vi "nanocal -- nuclear schottky fit V5.vi"() -> ()   [LabVIEW 2020] (continued)
__sam_\" ->   <|    \"ζ\" -> 0.023098882919   ,  \"τ1\" -> 0.017709986922   ,  \"τS\" -> 0.038881575014   ,  \"τN\" -> 0.000747654909   ,  \"τC\" -> 0.003803962289   ,  \"κ0\" -> 0.000000003538   ,  \"mm1\" -> 0.000078528513   ,  \"mm2\" -> 0.017209583260   ,  \"mm3\" -> 0.044770458303   ,  \"T\" -> 0.530000000000   ,  \"B\" -> 5.000000000000   ,  \"θ\" -> 90.000000000000   ,  \"Reoff\" -> -1599397.590361446140   ,  \"Imoff\" -> 0.000000000000    |>   , \r\"IDS0344_210904_RAW_cal__ref_\" ->   <|    \"ζ\" -> 0.030262302634   ,  \"τ1\" -> 0.017398280529   ,  \"τS\" -> 0.027078056707   ,  \"τN\" -> 0.000382363637   ,  \"τC\" -> 0.002680781698   ,  \"κ0\" -> 0.000000003878   ,  \"mm1\" -> 0.000072009464   ,  \"mm2\" -> 0.016908620237   ,  \"mm3\" -> 0.031389868421   ,  \"T\" -> 0.620000000000   ,  \"B\" -> 5.000000000000   ,  \"θ\" -> 90.000000000000   ,  \"Reoff\" -> -1891089.108910888430   ,  \"Imoff\" -> 0.000000000000    |>   , \r\"IDS0344_210904_RAW_cal__sam_\" ->   <|    \"ζ\" -> 0.019239644947   ,  \"τ1\" -> 0.016162010817   ,  \"τS\" -> 0.033688234899   ,  \"τN\" -> 0.000426792406   ,  \"τC\" -> 0.004393456024   ,  \"κ0\" -> 0.000000004224   ,  \"mm1\" -> 0.000073664779   ,  \"mm2\" -> 0.015859557336   ,  \"mm3\" -> 0.039393633044   ,  \"T\" -> 0.620000000000   ,  \"B\" -> 5.000000000000   ,  \"θ\" -> 90.000000000000   ,  \"Reoff\" -> -1105421.686746988450   ,  \"Imoff\" -> 0.000000000000    |>   , \r\"IDS0346_210904_RAW_cal__ref_\" ->   <|    \"ζ\" -> 0.393492726310   ,  \"τ1\" -> 0.048485470918   ,  \"τS\" -> 0.113472046437   ,  \"τN\" -> 0.239298779337   ,  \"τC\" -> 0.001078750584   ,  \"κ0\" -> 0.000000000381   ,  \"mm1\" -> 0.000303109396   ,  \"mm2\" -> 0.014642186944   ,  \"mm3\" -> 0.526202504932   ,  \"T\" -> 0.122000000000   ,  \"B\" -> 8.000000000000   ,  \"θ\" -> 90.000000000000   ,  \"Reoff\" -> -154102409.638554215000   ,  \"Imoff\" -> 0.000000000000    |>   , \r\"IDS0346_210904_RAW_cal__sam_\" ->   <|    \"ζ\" -> 0.199267253863   ,  \"τ1\" -> 0.050205114691   ,  \"τS\" -> 0.125855812683   ,  \"τN\" -> 0.296749666016   ,  \"τC\" -> 0.001624351903   ,  \"κ0\" -> 0.000000000535   ,  \"mm1\" -> 0.000267463038   ,  \"mm2\" -> 0.014047868056   ,  \"mm3\" -> 0.544331047407   ,  \"T\" -> 0.122000000000   ,  \"B\" -> 8.000000000000   ,  \"θ\" -> 90.000000000000   ,  \"Reoff\" -> -35716867.469879508000   ,  \"Imoff\" -> 0.000000000000    |>   , \r\"IDS0347_210906_RAW_cal__ref_\" ->   <|    \"ζ\" -> 0.286601830164   ,  \"τ1\" -> 0.041889464943   ,  \"τS\" -> 0.071636933344   ,  \"τN\" -> 0.093950517978   ,  \"τC\" -> 0.001090880876   ,  \"κ0\" -> 0.000000000643   ,  \"mm1\" -> 0.000240765602   ,  \"mm2\" -> 0.016269353914   ,  \"mm3\" -> 0.239515344226   ,  \"T\" -> 0.157000000000   ,  \"B\" -> 8.000000000000   ,  \"θ\" -> 90.000000000000   ,  \"Reoff\" -> -67247524.752475246800   ,  \"Imoff\" -> 0.000000000000    |>   , \r\"IDS0347_210906_RAW_cal__sam_\" ->   <|    \"ζ\" -> 0.169709128246   ,  \"τ1\" -> 0.042569783210   ,  \"τS\" -> 0.096466158196   ,  \"τN\" -> 0.116379310482   ,  \"τC\" -> 0.001498996005   ,  \"κ0\" -> 0.000000000766   ,  \"mm1\" -> 0.000215022431   ,  \"mm2\" -> 0.017656553883   ,  \"mm3\" -> 0.275164490520   ,  \"T\" -> 0.157000000000   ,  \"B\" -> 8.000000000000   ,  \"θ\" -> 90.000000000000   ,  \"Reoff\" -> -35716867.469879508000   ,  \"Imoff\" -> 0.000000000000    |>   , \r\"IDS0348_210906_RAW_cal__ref_\" ->   <|    \"ζ\" -> 0.227729495252   ,  \"τ1\" -> 0.036551248252   ,  \"τS\" -> 0.056246960900   ,  \"τN\" -> 0.064010200838   ,  \"τC\" -> 0.001130245474   ,  \"κ0\" -> 0.000000000764   ,  \"mm1\" -> 0.000206863244   ,  \"mm2\" -> 0.015040543137   ,  \"mm3\" -> 0.170077351826   ,  \"T\" -> 0.178000000000   ,  \"B\" -> 8.000000000000   ,  \"θ\" -> 90.000000000000   ,  \"Reoff\" -> -42981927.710843384300   ,  \"Imoff\" -> 0.000000000000    |>   , \r\"IDS0348_210906_RAW_cal__sam_\" ->   <|    \"ζ\" -> 0.135783247929   ,  \"τ1\" -> 0.037121050091   ,  \"τS\" -> 0.079201640502   ,  \"τN\" -> 0.079201640502   ,  \"τC\" -> 0.001474311209   ,  \"κ0\" -> 0.000000000894   ,  \"mm1\" -> 0.000173730712   ,  \"mm2\" -> 0.016810842330   ,  \"mm3\" -> 0.201522581240   ,  \"T\" -> 0.178000000000   ,  \"B\" -> 8.000000000000   ,  \"θ\" -> 90.000000000000   ,  \"Reoff\" -> -29680722.891566276600   ,  \"Imoff\" -> 0.000000000000    |>   , \r\"IDS0349_210906_RAW_cal__ref_\" ->   <|    \"ζ\" -> 0.192717199831   ,  \"τ1\" -> 0.031244125663   ,  \"τS\" -> 0.051644649093   ,  \"τN\" -> 0.037139184979   ,  \"τC\" -> 0.001129392389   ,  \"κ0\" -> 0.000000001033   ,  \"mm1\" -> 0.000179703108   ,  \"mm2\" -> 0.016008954190   ,  \"mm3\" -> 0.122078866718   ,  \"T\" -> 0.200000000000   ,  \"B\" -> 8.000000000000   ,  \"θ\" -> 90.000000000000   ,  \"Reoff\" -> -27280120.481927722700   ,  \"Imoff\" -> 0.000000000000    |>   , \r\"IDS0349_210906_RAW_cal__sam_\" ->   <|    \"ζ\" -> 0.113690190882   ,  \"τ1\" -> 0.032691214581   ,  \"τS\" -> 0.068786957350   ,  \"τN\" -> 0.048058332081   ,  \"τC\" -> 0.001613875480   ,  \"κ0\" -> 0.000000001156   ,  \"mm1\" -> 0.000161675745   ,  \"mm2\" -> 0.017372504664   ,  \"mm3\" -> 0.146900362342   ,  \"T\" -> 0.200000000000   ,  \"B\" -> 8.000000000000   ,  \"θ\" -> 90.000000000000   ,  \"Reoff\" -> -14590361.445783138300   ,  \"Imoff\" -> 0.000000000000    |>   , \r\"IDS0350_210906_RAW_cal__ref_\" ->   <|    \"ζ\" -> 0.118307141768   ,  \"τ1\" -> 0.026492736989   ,  \"τS\" -> 0.042057283761   ,  \"τN\" -> 0.016294526354   ,  \"τC\" -> 0.001283997162   ,  \"κ0\" -> 0.000000001348   ,  \"mm1\" -> 0.000132583586   ,  \"mm2\" -> 0.016768408652   ,  \"mm3\" -> 0.076130987900   ,  \"T\" -> 0.260000000000   ,  \"B\" -> 8.000000000000   ,  \"θ\" -> 90.000000000000   ,  \"Reoff\" -> -15307228.915662650000   ,  \"Imoff\" -> 0.000000000000    |>   , \r\"IDS0350_210906_RAW_cal__sam_\" ->   <|    \"ζ\" -> 0.071614468485   ,  \"τ1\" -> 0.024327525692   ,  \"τS\" -> 0.055056024171   ,  \"τN\" -> 0.019709093999   ,  \"τC\" -> 0.001754398678   ,  \"κ0\" -> 0.000000001497   ,  \"mm1\" -> 0.000114067222   ,  \"mm2\" -> 0.016460052715   ,  \"mm3\" -> 0.089627186802   ,  \"T\" -> 0.260000000000   ,  \"B\" -> 8.000000000000   ,  \"θ\" -> 90.000000000000   ,  \"Reoff\" -> -10063253.012048184900   ,  \"Imoff\" -> 0.000000000000    |>   , \r\"IDS0351_210906_RAW_cal__ref_\" ->   <|    \"ζ\" -> 0.080949504792   ,  \"τ1\" -> 0.020979423468   ,  \"τS\" -> 0.037020600701   ,  \"τN\" -> 0.007895851637   ,  \"τC\" -> 0.001560889580   ,  \"κ0\" -> 0.000000001762   ,  \"mm1\" -> 0.000112804280   ,  \"mm2\" -> 0.015752171207   ,  \"mm3\" -> 0.055227754472   ,  \"T\" -> 0.310000000000   ,  \"B\" -> 8.000000000000   ,  \"θ\" -> 90.000000000000   ,  \"Reoff\" -> -7470297.029702961450   ,  \"Imoff\" -> 0.000000000000    |>   , \r\"IDS0351_210906_RAW_cal__sam_\" ->   <|    \"ζ\" -> 0.049866383839   ,  \"τ1\" -> 0.023285662985   ,  \"τS\" -> 0.049370833464   ,  \"τN\" -> 0.009866658615   ,  \"τC\" -> 0.002153040267   ,  \"κ0\" -> 0.000000001928   ,  \"mm1\" -> 0.000098362318   ,  \"mm2\" -> 0.018063601956   ,  \"mm3\" -> 0.069468190575   ,  \"T\" -> 0.310000000000   ,  \"B\" -> 8.000000000000   ,  \"θ\" -> 90.000000000000   ,  \"Reoff\" -> -5536144.578313261270   ,  \"Imoff\" -> 0.000000000000    |>   , \r\"IDS0352_210906_RAW_cal__ref_\" ->   <|    \"ζ\" -> 0.059925182504   ,  \"τ1\" -> 0.020454762932   ,  \"τS\" -> 0.034343460335   ,  \"τN\" -> 0.004837229977   ,  \"τC\" -> 0.001951906105   ,  \"κ0\" -> 0.000000002109   ,  \"mm1\" -> 0.000105022903   ,  \"mm2\" -> 0.016546778145   ,  \"mm3\" -> 0.047283468319   ,  \"T\" -> 0.360000000000   ,  \"B\" -> 8.000000000000   ,  \"θ\" -> 90.000000000000   ,  \"Reoff\" -> -3485148.514851480720   ,  \"Imoff\" -> 0.000000000000    |>   , \r\"IDS0352_210906_RAW_cal__sam_\" ->   <|    \"ζ\" -> 0.036116393265   ,  \"τ1\" -> 0.020310974732   ,  \"τS\" -> 0.044594628397   ,  \"τN\" -> 0.005932938101   ,  \"τC\" -> 0.002747123875   ,  \"κ0\" -> 0.000000002292   ,  \"mm1\" -> 0.000090548575   ,  \"mm2\" -> 0.017024776182   ,  \"mm3\" -> 0.058295213810   ,  \"T\" -> 0.360000000000   ,  \"B\" -> 8.000000000000   ,  \"θ\" -> 90.000000000000   ,  \"Reoff\" -> -2518072.289156645540   ,  \"Imoff\" -> 0.000000000000    |>   , \r\"IDS0353_210906_RAW_cal__ref_\" ->   <|    \"ζ\" -> 0.045101316453   ,  \"τ1\" -> 0.020505895958   ,  \"τS\" -> 0.031209032196   ,  \"τN\" -> 0.002683750708   ,  \"τC\" -> 0.002226651105   ,  \"κ0\" -> 0.000000002626   ,  \"mm1\" -> 0.000090181690   ,  \"mm2\" -> 0.017621773769   ,  \"mm3\" -> 0.040441983634   ,  \"T\" -> 0.438000000000   ,  \"B\" -> 8.000000000000   ,  \"θ\" -> 90.000000000000   ,  \"Reoff\" -> -2688118.811881184580   ,  \"Imoff\" -> 0.000000000000    |>   , \r\"IDS0353_210906_RAW_cal__sam_\" ->   <|    \"ζ\" -> 0.028235631162   ,  \"τ1\" -> 0.018033623612   ,  \"τS\" -> 0.040112967891   ,  \"τN\" -> 0.003332308168   ,  \"τC\" -> 0.002994357278   ,  \"κ0\" -> 0.000000002859   ,  \"mm1\" -> 0.000076791949   ,  \"mm2\" -> 0.016073609718   ,  \"mm3\" -> 0.049549560072   ,  \"T\" -> 0.438000000000   ,  \"B\" -> 8.000000000000   ,  \"θ\" -> 90.000000000000   ,  \"Reoff\" -> -2200000.000000000000   ,  \"Imoff\" -> 0.000000000000    |>   , \r\"IDS0354_210906_RAW_cal__ref_\" ->   <|    \"ζ\" -> 0.035437454716   ,  \"τ1\" -> 0.018601112933   ,  \"τS\" -> 0.028168170851   ,  \"τN\" -> 0.001514485444   ,  \"τC\" -> 0.002620014428   ,  \"κ0\" -> 0.000000003276   ,  \"mm1\" -> 0.000082490473   ,  \"mm2\" -> 0.016827947950   ,  \"mm3\" -> 0.035045223022   ,  \"T\" -> 0.530000000000   ,  \"B\" -> 8.000000000000   ,  \"θ\" -> 90.000000000000   ,  \"Reoff\" -> -2000000.000000000000   ,  \"Imoff\" -> 0.000000000000    |>   , \r\"IDS0354_210906_RAW_cal__sam_\" ->   <|    \"ζ\" -> 0.022962333090   ,  \"τ1\" -> 0.020865157142   ,  \"τS\" -> 0.035948400917   ,  \"τN\" -> 0.001990138096   ,  \"τC\" -> 0.003574397791   ,  \"κ0\" -> 0.000000003542   ,  \"mm1\" -> 0.000073258085   ,  \"mm2\" -> 0.019040364220   ,  \"mm3\" -> 0.044135629011   ,  \"T\" -> 0.530000000000   ,  \"B\" -> 8.000000000000   ,  \"θ\" -> 90.000000000000   ,  \"Reoff\" -> -1700000.000000000000   ,  \"Imoff\" -> 0.000000000000    |>   , \r\"IDS0355_210906_RAW_cal__ref_\" ->   <|    \"ζ\" -> 0.022657414888   ,  \"τ1\" -> 0.018817554935   ,  \"τS\" -> 0.021193839370   ,  \"τN\" -> 0.000511146216   ,  \"τC\" -> 0.003920154705   ,  \"κ0\" -> 0.000000005412   ,  \"mm1\" -> 0.000073761374   ,  \"mm2\" -> 0.017646851698   ,  \"mm3\" -> 0.027213861018   ,  \"T\" -> 0.830000000000   ,  \"B\" -> 8.000000000000   ,  \"θ\" -> 90.000000000000   ,  \"Reoff\" -> -695544.554455444216   ,  \"Imoff\" -> 0.000000000000    |>   , \r\"IDS0355_210906_RAW_cal__sam_\" ->   <|    \"ζ\" -> 0.015987398390   ,  \"τ1\" -> 0.023974349678   ,  \"τS\" -> 0.025824294014   ,  \"τN\" -> 0.000573136357   ,  \"τC\" -> 0.005688548480   ,  \"κ0\" -> 0.000000005865   ,  \"mm1\" -> 0.000073733721   ,  \"mm2\" -> 0.022561297233   ,  \"mm3\" -> 0.033847323811   ,  \"T\" -> 0.830000000000   ,  \"B\" -> 8.000000000000   ,  \"θ\" -> 90.000000000000   ,  \"Reoff\" -> -599999.999999999999   ,  \"Imoff\" -> 0.000000000000    |>   , \r\"IDS0359_210907_RAW_cal__ref_\" ->   <|    \"ζ\" -> 0.381003010305   ,  \"τ1\" -> 0.094337322163   ,  \"τS\" -> 0.076926495749   ,  \"τN\" -> 0.550745531665   ,  \"τC\" -> 0.001029575567   ,  \"κ0\" -> 0.000000000382   ,  \"mm1\" -> 0.000282020135   ,  \"mm2\" -> 0.010610910676   ,  \"mm3\" -> 0.951290926262   ,  \"T\" -> 0.120000000000   ,  \"B\" -> 12.000000000000   ,  \"θ\" -> 60.000000000000   ,  \"Reoff\" -> -100000000.000000000000   ,  \"Imoff\" -> 0.000000000000    |>   , \r\"IDS0359_210907_RAW_cal__sam_\" ->   <|    \"ζ\" -> 0.241762987309   ,  \"τ1\" -> 0.090301757431   ,  \"τS\" -> 0.104468976957   ,  \"τN\" -> 0.810352557873   ,  \"τC\" -> 0.001702208121   ,  \"κ0\" -> 0.000000000500   ,  \"mm1\" -> 0.000327834342   ,  \"mm2\" -> 0.009723084216   ,  \"mm3\" -> 1.217944568939   ,  \"T\" -> 0.120000000000   ,  \"B\" -> 12.000000000000   ,  \"θ\" -> 60.000000000000   ,  \"Reoff\" -> -52289156.626506023100   ,  \"Imoff\" -> 0.000000000000    |>   , \r\"IDS0360_210907_RAW_cal__ref_\" ->   <|    \"ζ\" -> 0.332195625520   ,  \"τ1\" -> 0.077786303593   ,  \"τS\" -> 0.054222210065   ,  \"τN\" -> 0.276486324199   ,  \"τC\" -> 0.001063947875   ,  \"κ0\" -> 0.000000000641   ,  \"mm1\" -> 0.000262343099   ,  \"mm2\" -> 0.011186309949   ,  \"mm3\" -> 0.507970061088   ,  \"T\" -> 0.150000000000   ,  \"B\" -> 12.000000000000   ,  \"θ\" -> 60.000000000000   ,  \"Reoff\" -> -64885542.168674700000   ,  \"Imoff\" -> 0.000000000000    |>   , \r\"IDS0360_210907_RAW_cal__sam_\" ->   <|    \"ζ\" -> 0.201278537585   ,  \"τ1\" -> 0.081544073952   ,  \"τS\" -> 0.088995303529   ,  \"τN\" -> 0.405130496924   ,  \"τC\" -> 0.001460686320   ,  \"κ0\" -> 0.000000000739   ,  \"mm1\" -> 0.000241947199   ,  \"mm2\" -> 0.013299947862   ,  \"mm3\" -> 0.663045584163   ,  \"T\" -> 0.150000000000   ,  \"B\" -> 12.000000000000   ,  \"θ\" -> 60.000000000000   ,  \"Reoff\" -> -39048192.771084338400   ,  \"Imoff\" -> 0.000000000000    |>   , \r\"IDS0361_210908_RAW_cal__ref_\" ->   <|    \"ζ\" -> 0.279940228007   ,  \"τ1\" -> 0.067057240536   ,  \"τS\" -> 0.048025817643   ,  \"τN\" -> 0.170011495172   ,  \"τC\" -> 0.001015047914   ,  \"κ0\" -> 0.000000000754   ,  \"mm1\" -> 0.000219134041   ,  \"mm2\" -> 0.012486551439   ,  \"mm3\" -> 0.334441330849   ,  \"T\" -> 0.168000000000   ,  \"B\" -> 12.000000000000   ,  \"θ\" -> 60.000000000000   ,  \"Reoff\" -> 0.000000000000   ,  \"Imoff\" -> 0.000000000000    |>   , \r\"IDS0361_210908_RAW_cal__sam_\" ->   <|    \"ζ\" -> 0.166104690940   ,  \"τ1\" -> 0.071049175548   ,  \"τS\" -> 0.068661809155   ,  \"τN\" -> 0.222482953546   ,  \"τC\" -> 0.001364223445   ,  \"κ0\" -> 0.000000000861   ,  \"mm1\" -> 0.000191495940   ,  \"mm2\" -> 0.014533832786   ,  \"mm3\" -> 0.397193343795   ,  \"T\" -> 0.168000000000   ,  \"B\" -> 12.000000000000   ,  \"θ\" -> 60.000000000000   ,  \"Reoff\" -> -34789156.626506023100   ,  \"Imoff\" -> 0.000000000000    |>   , \r\"IDS0362_210908_RAW_cal__ref_\" ->   <|    \"ζ\" -> 0.206594976212   ,  \"τ1\" -> 0.057885925979   ,  \"τS\" -> 0.038698575169   ,  \"τN\" -> 0.092347634602   ,  \"τC\" -> 0.001108131545   ,  \"κ0\" -> 0.000000001046   ,  \"mm1\" -> 0.000186033666   ,  \"mm2\" -> 0.013554841704   ,  \"mm3\" -> 0.203372880515   ,  \"T\" -> 0.197000000000   ,  \"B\" -> 12.000000000000   ,  \"θ\" -> 60.000000000000   ,  \"Reoff\" -> 0.000000000000   ,  \"Imoff\" -> 0.000000000000    |>   , \r\"IDS0362_210908_RAW_cal__sam_\" ->   <|    \"ζ\" -> 0.123741217510   ,  \"τ1\" -> 0.059103977068   ,  \"τS\" -> 0.051096152058   ,  \"τN\" -> 0.122661863704   ,  \"τC\" -> 0.001502836172   ,  \"κ0\" -> 0.000000001149   ,  \"mm1\" -> 0.000161683871   ,  \"mm2\" -> 0.014394250129   ,  \"mm3\" -> 0.241309923424   ,  \"T\" -> 0.197000000000   ,  \"B\" -> 12.000000000000   ,  \"θ\" -> 60.000000000000   ,  \"Reoff\" -> -17448795.180722892300   ,  \"Imoff\" -> 0.000000000000    |>   , \r\"IDS0363_210908_RAW_cal__ref_\" ->   <|    \"ζ\" -> 0.123216898961   ,  \"τ1\" -> 0.041424716624   ,  \"τS\" -> 0.030606562009   ,  \"τN\" -> 0.033679175657   ,  \"τC\" -> 0.001245281919   ,  \"κ0\" -> 0.000000001353   ,  \"mm1\" -> 0.000132308811   ,  \"mm2\" -> 0.014696535073   ,  \"mm3\" -> 0.100047981568   ,  \"T\" -> 0.250000000000   ,  \"B\" -> 12.000000000000   ,  \"θ\" -> 60.000000000000   ,  \"Reoff\" -> 0.000000000000   ,  \"Imoff\" -> 0.000000000000    |>   , \r\"IDS0363_210908_RAW_cal__sam_\" ->   <|    \"ζ\" -> 0.074359211271   ,  \"τ1\" -> 0.044477620306   ,  \"τS\" -> 0.040449563551   ,  \"τN\" -> 0.044745540249   ,  \"τC\" -> 0.001712765821   ,  \"κ0\" -> 0.000000001493   ,  \"mm1\" -> 0.000114327803   ,  \"mm2\" -> 0.016556677808   ,  \"mm3\" -> 0.121049525039   ,  \"T\" -> 0.250000000000   ,  \"B\" -> 12.000000000000   ,  \"θ\" -> 60.000000000000   ,  \"Reoff\" -> -10147590.361445784600   ,  \"Imoff\" -> 0.000000000000    |>   , \r\"IDS0364_210908_RAW_cal__ref_\" ->   <|    \"ζ\" -> 0.083979493288   ,  \"τ1\" -> 0.035863468022   ,  \"τS\" -> 0.027413945050   ,  \"τN\" -> 0.017174500536   ,  \"τC\" -> 0.001551957186   ,  \"κ0\" -> 0.000000001738   ,  \"mm1\" -> 0.000114677510   ,  \"mm2\" -> 0.016060377955   ,  \"mm3\" -> 0.069573330396   ,  \"T\" -> 0.307000000000   ,  \"B\" -> 12.000000000000   ,  \"θ\" -> 60.000000000000   ,  \"Reoff\" -> 0.000000000000   ,  \"Imoff\" -> 0.000000000000    |>   , \r\"IDS0364_210908_RAW_cal__sam_\" ->   <|    \"ζ\" -> 0.051560123380   ,  \"τ1\" -> 0.037167172913   ,  \"τS\" -> 0.035875072163   ,  \"τN\" -> 0.021782945969   ,  \"τC\" -> 0.002191662682   ,  \"κ0\" -> 0.000000001902   ,  \"mm1\" -> 0.000101812126   ,  \"mm2\" -> 0.018093196790   ,  \"mm3\" -> 0.081794699340   ,  \"T\" -> 0.307000000000   ,  \"B\" -> 12.000000000000   ,  \"θ\" -> 60.000000000000   ,  \"Reoff\" -> -5584337.349397592250   ,  \"Imoff\" -> 0.000000000000    |>   , \r\"IDS0365_210908_RAW_cal__ref_\" ->   <|    \"ζ\" -> 0.061526991224   ,  \"τ1\" -> 0.029624261727   ,  \"τS\" -> 0.025208021627   ,  \"τN\" -> 0.009698502183   ,  \"τC\" -> 0.001918212332   ,  \"κ0\" -> 0.000000002116   ,  \"mm1\" -> 0.000104113340   ,  \"mm2\" -> 0.016183109270   ,  \"mm3\" -> 0.052309468643   ,  \"T\" -> 0.360000000000   ,  \"B\" -> 12.000000000000   ,  \"θ\" -> 60.000000000000   ,  \"Reoff\" -> 0.000000000000   ,  \"Imoff\" -> 0.000000000000    |>   , \r\"IDS0365_210908_RAW_cal__sam_\" ->   <|    \"ζ\" -> 0.037527154631   ,  \"τ1\" -> 0.031791574880   ,  \"τS\" -> 0.032568278603   ,  \"τN\" -> 0.012463984296   ,  \"τC\" -> 0.002682405917   ,  \"κ0\" -> 0.000000002306   ,  \"mm1\" -> 0.000090102201   ,  \"mm2\" -> 0.018466994147   ,  \"mm3\" -> 0.062639080041   ,  \"T\" -> 0.360000000000   ,  \"B\" -> 12.000000000000   ,  \"θ\" -> 60.000000000000   ,  \"Reoff\" -> -2846385.542168676850   ,  \"Imoff\" -> 0.000000000000    |>   , \r\"IDS0366_210908_RAW_cal__ref_\" ->   <|    \"ζ\" -> 0.045515267447   ,  \"τ1\" -> 0.026001810196   ,  \"τS\" -> 0.023136668780   ,  \"τN\" -> 0.005224117981   ,  \"τC\" -> 0.002327400857   ,  \"κ0\" -> 0.000000002646   ,  \"mm1\" -> 0.000092745821   ,  \"mm2\" -> 0.016670952378   ,  \"mm3\" -> 0.041217148409   ,  \"T\" -> 0.430000000000   ,  \"B\" -> 12.000000000000   ,  \"θ\" -> 60.000000000000   ,  \"Reoff\" -> 0.000000000000   ,  \"Imoff\" -> 0.000000000000    |>   , \r\"IDS0366_210908_RAW_cal__sam_\" ->   <|    \"ζ\" -> 0.029143715364   ,  \"τ1\" -> 0.026198855926   ,  \"τS\" -> 0.029745373312   ,  \"τN\" -> 0.006649011545   ,  \"τC\" -> 0.003090491846   ,  \"κ0\" -> 0.000000002869   ,  \"mm1\" -> 0.000079676072   ,  \"mm2\" -> 0.018163106475   ,  \"mm3\" -> 0.048501617675   ,  \"T\" -> 0.430000000000   ,  \"B\" -> 12.000000000000   ,  \"θ\" -> 60.000000000000   ,  \"Reoff\" -> -2237951.807228915390   ,  \"Imoff\" -> 0.000000000000    |>   , \r\"IDS0367_210908_RAW_cal__ref_\" ->   <|    \"ζ\" -> 0.037324451442   ,  \"τ1\" -> 0.019605264024   ,  \"τS\" -> 0.021700560504   ,  \"τN\" -> 0.002800944156   ,  \"τC\" -> 0.002526998509   ,  \"κ0\" -> 0.000000003301   ,  \"mm1\" -> 0.000082012466   ,  \"mm2\" -> 0.015132192259   ,  \"mm3\" -> 0.032334067689   ,  \"T\" -> 0.530000000000   ,  \"B\" -> 12.000000000000   ,  \"θ\" -> 60.000000000000   ,  \"Reoff\" -> 0.000000000000   ,  \"Imoff\" -> 0.000000000000    |>   , \r\"IDS0367_210908_RAW_cal__sam_\" ->   <|    \"ζ\" -> 0.024637271207   ,  \"τ1\" -> 0.025634847148   ,  \"τS\" -> 0.027302474030   ,  \"τN\" -> 0.003538185279   ,  \"τC\" -> 0.003933377133   ,  \"κ0\" -> 0.000000003566   ,  \"mm1\" -> 0.000083131278   ,  \"mm2\" -> 0.019726981228   ,  \"mm3\" -> 0.041358600771   ,  \"T\" -> 0.530000000000   ,  \"B\" -> 12.000000000000   ,  \"θ\" -> 60.000000000000   ,  \"Reoff\" -> -1629518.072289161380   ,  \"Imoff\" -> 0.000000000000    |>   , \r\"IDS0368_210908_RAW_cal__ref_\" ->   <|    \"ζ\" -> 0.030581023885   ,  \"τ1\" -> 0.017326525290   ,  \"τS\" -> 0.020225378130   ,  \"τN\" -> 0.001703135365   ,  \"τC\" -> 0.003380889395   ,  \"κ0\" -> 0.000000003914   ,  \"mm1\" -> 0.000086626446   ,  \"mm2\" -> 0.014628874360   ,  \"mm3\" -> 0.028591023770   ,  \"T\" -> 0.630000000000   ,  \"B\" -> 12.000000000000   ,  \"θ\" -> 60.000000000000   ,  \"Reoff\" -> 0.000000000000   ,  \"Imoff\" -> 0.000000000000    |>   , \r\"IDS0368_210908_RAW_cal__sam_\" ->   <|    \"ζ\" -> 0.021420270760   ,  \"τ1\" -> 0.018208454683   ,  \"τS\" -> 0.024985612374   ,  \"τN\" -> 0.002144760910   ,  \"τC\" -> 0.004931614434   ,  \"κ0\" -> 0.000000004254   ,  \"mm1\" -> 0.000086915042   ,  \"mm2\" -> 0.015826314138   ,  \"mm3\" -> 0.034938353162   ,  \"T\" -> 0.630000000000   ,  \"B\" -> 12.000000000000   ,  \"θ\" -> 60.000000000000   ,  \"Reoff\" -> -1204819.277108438310   ,  \"Imoff\" -> 0.000000000000    |>   , \r\"IDS0369_210908_RAW_cal__ref_\" ->   <|    \"ζ\" -> 0.022212344829   ,  \"τ1\" -> 0.017343641344   ,  \"τS\" -> 0.018001662092   ,  \"τN\" -> 0.000711569404   ,  \"τC\" -> 0.004309595418   ,  \"κ0\" -> 0.000000005439   ,  \"mm1\" -> 0.000076128819   ,  \"mm2\" -> 0.015699102017   ,  \"mm3\" -> 0.025006902173   ,  \"T\" -> 0.830000000000   ,  \"B\" -> 12.000000000000   ,  \"θ\" -> 60.000000000000   ,  \"Reoff\" -> 0.000000000000   ,  \"Imoff\" -> 0.000000000000    |>   , \r\"IDS0369_210908_RAW_cal__sam_\" ->   <|    \"ζ\" -> 0.014606512986   ,  \"τ1\" -> 0.019756664879   ,  \"τS\" -> 0.022303249954   ,  \"τN\" -> 0.001023812506   ,  \"τC\" -> 0.005490022400   ,  \"κ0\" -> 0.000000005866   ,  \"mm1\" -> 0.000063747249   ,  \"mm2\" -> 0.017921258799   ,  \"mm3\" -> 0.030929470731   ,  \"T\" -> 0.830000000000   ,  \"B\" -> 12.000000000000   ,  \"θ\" -> 60.000000000000   ,  \"Reoff\" -> -481927.710843376814   ,  \"Imoff\" -> 0.000000000000    |>   , \r\"IDS0370_210908_RAW_cal__ref_\" ->   <|    \"ζ\" -> 0.021569402950   ,  \"τ1\" -> 0.017921737944   ,  \"τS\" -> 0.015463128015   ,  \"τN\" -> 0.000390873619   ,  \"τC\" -> 0.004954240411   ,  \"κ0\" -> 0.000000007586   ,  \"mm1\" -> 0.000079935600   ,  \"mm2\" -> 0.016393641357   ,  \"mm3\" -> 0.022598364382   ,  \"T\" -> 1.130000000000   ,  \"B\" -> 12.000000000000   ,  \"θ\" -> 60.000000000000   ,  \"Reoff\" -> 0.000000000000   ,  \"Imoff\" -> 0.000000000000    |>   , \r\"IDS0370_210908_RAW_cal__sam_\" ->   <|    \"ζ\" -> 0.013427569249   ,  \"τ1\" -> 0.019934074843   ,  \"τS\" -> 0.019524726442   ,  \"τN\" -> 0.000513623253   ,  \"τC\" -> 0.005657316251   ,  \"κ0\" -> 0.000000008143   ,  \"mm1\" -> 0.000058424467   ,  \"mm2\" -> 0.018528796956   ,  \"mm3\" -> 0.027311585694   ,  \"T\" -> 1.130000000000   ,  \"B\" -> 12.000000000000   ,  \"θ\" -> 60.000000000000   ,  \"Reoff\" -> -481927.710843376814   ,  \"Imoff\" -> 0.000000000000    |>   , \r\"IDS0371_210908_RAW_cal__ref_\" ->   <|    \"ζ\" -> 0.020664849580   ,  \"τ1\" -> 0.018108723176   ,  \"τS\" -> 0.010299896170   ,  \"τN\" -> 0.000079818017   ,  \"τC\" -> 0.006259144045   ,  \"κ0\" -> 0.000000013130   ,  \"mm1\" -> 0.000079811267   ,  \"mm2\" -> 0.016056535433   ,  \"mm3\" -> 0.018825729941   ,  \"T\" -> 1.900000000000   ,  \"B\" -> 12.000000000000   ,  \"θ\" -> 60.000000000000   ,  \"Reoff\" -> 0.000000000000   ,  \"Imoff\" -> 0.000000000000    |>   , \r\"IDS0371_210908_RAW_cal__sam_\" ->   <|    \"ζ\" -> 0.009645933094   ,  \"τ1\" -> 0.020976887035   ,  \"τS\" -> 0.013140254521   ,  \"τN\" -> 0.000215522697   ,  \"τC\" -> 0.007317042194   ,  \"κ0\" -> 0.000000013897   ,  \"mm1\" -> 0.000045154509   ,  \"mm2\" -> 0.018728618799   ,  \"mm3\" -> 0.023004762073   ,  \"T\" -> 1.900000000000   ,  \"B\" -> 12.000000000000   ,  \"θ\" -> 60.000000000000   ,  \"Reoff\" -> -120481.927710846066   ,  \"Imoff\" -> 0.000000000000    |>   , \r\"IDS0372_210908_RAW_cal__ref_\" ->   <|    \"ζ\" -> 0.021592146431   ,  \"τ1\" -> 0.018093446545   ,  \"τS\" -> 0.007071841556   ,  \"τN\" -> 0.000029085223   ,  \"τC\" -> 0.005341206531   ,  \"κ0\" -> 0.000000023517   ,  \"mm1\" -> 0.000065243548   ,  \"mm2\" -> 0.012435446609   ,  \"mm3\" -> 0.018188213949   ,  \"T\" -> 3.110000000000   ,  \"B\" -> 12.000000000000   ,  \"θ\" -> 60.000000000000   ,  \"Reoff\" -> 0.000000000000   ,  \"Imoff\" -> 0.000000000000    |>   , \r\"IDS0372_210908_RAW_cal__sam_\" ->   <|    \"ζ\" -> 0.010006554735   ,  \"τ1\" -> 0.021193289022   ,  \"τS\" -> 0.010059776467   ,  \"τN\" -> 0.000092737128   ,  \"τC\" -> 0.005619947239   ,  \"κ0\" -> 0.000000024358   ,  \"mm1\" -> 0.000035931477   ,  \"mm2\" -> 0.015490366222   ,  \"mm3\" -> 0.021541043840   ,  \"T\" -> 3.110000000000   ,  \"B\" -> 12.000000000000   ,  \"θ\" -> 60.000000000000   ,  \"Reoff\" -> -120481.927710846066   ,  \"Imoff\" -> 0.000000000000    |>   , \r\"IDS0373_210908_RAW_cal__ref_\" ->   <|    \"ζ\" -> 0.028148688120   ,  \"τ1\" -> 0.012706961955   ,  \"τS\" -> 0.003881518121   ,  \"τN\" -> 0.000007160132   ,  \"τC\" -> 0.004346615253   ,  \"κ0\" -> 0.000000058313   ,  \"mm1\" -> 0.000057355729   ,  \"mm2\" -> 0.008266435527   ,  \"mm3\" -> 0.012727925396   ,  \"T\" -> 5.750000000000   ,  \"B\" -> 12.000000000000   ,  \"θ\" -> 60.000000000000   ,  \"Reoff\" -> 0.000000000000   ,  \"Imoff\" -> 0.000000000000    |>   , \r\"IDS0373_210908_RAW_cal__sam_\" ->   <|    \"ζ\" -> 0.009383547393   ,  \"τ1\" -> 0.021616814113   ,  \"τS\" -> 0.006389723126   ,  \"τN\" -> 0.000031102862   ,  \"τC\" -> 0.004593168461   ,  \"κ0\" -> 0.000000059183   ,  \"mm1\" -> 0.000024995592   ,  \"mm2\" -> 0.010985466166   ,  \"mm3\" -> 0.021680596929   ,  \"T\" -> 5.750000000000   ,  \"B\" -> 12.000000000000   ,  \"θ\" -> 60.000000000000   ,  \"Reoff\" -> -40000.000000000000   ,  \"Imoff\" -> 0.000000000000    |>   , \r\"IDS0377_210909_RAW_cal__ref_\" ->   <|    \"ζ\" -> 0.219438770438   ,  \"τ1\" -> 0.080681392218   ,  \"τS\" -> 0.035040622968   ,  \"τN\" -> 0.027652400569   ,  \"τC\" -> 0.001058893563   ,  \"κ0\" -> 0.000000001039   ,  \"mm1\" -> 0.000186730204   ,  \"mm2\" -> 0.026816671944   ,  \"mm3\" -> 0.131187187170   ,  \"T\" -> 0.197000000000   ,  \"B\" -> 8.000000000000   ,  \"θ\" -> 0.000000000000   ,  \"Reoff\" -> -30030120.481927715200   ,  \"Imoff\" -> 0.000000000000    |>   , \r\"IDS0377_210909_RAW_cal__sam_\" ->   <|    \"ζ\" -> 0.135798490691   ,  \"τ1\" -> 0.079257563336   ,  \"τS\" -> 0.046440970443   ,  \"τN\" -> 0.031537801980   ,  \"τC\" -> 0.001434159670   ,  \"κ0\" -> 0.000000001166   ,  \"mm1\" -> 0.000167444282   ,  \"mm2\" -> 0.031002991367   ,  \"mm3\" -> 0.138089459380   ,  \"T\" -> 0.197000000000   ,  \"B\" -> 8.000000000000   ,  \"θ\" -> 0.000000000000   ,  \"Reoff\" -> -18665662.650602411500   ,  \"Imoff\" -> 0.000000000000    |>   , \r\"IDS0378_210909_RAW_cal__ref_\" ->   <|    \"ζ\" -> 0.442149990737   ,  \"τ1\" -> 0.131337022654   ,  \"τS\" -> 0.122153878888   ,  \"τN\" -> 0.148135837540   ,  \"τC\" -> 0.001228213968   ,  \"κ0\" -> 0.000000000395   ,  \"mm1\" -> 0.000374737323   ,  \"mm2\" -> 0.049172044122   ,  \"mm3\" -> 0.472816767221   ,  \"T\" -> 0.122000000000   ,  \"B\" -> 8.000000000000   ,  \"θ\" -> 0.000000000000   ,  \"Reoff\" -> -103762048.192771077000   ,  \"Imoff\" -> 0.000000000000    |>   , \r\"IDS0378_210909_RAW_cal__sam_\" ->   <|    \"ζ\" -> 0.261650469875   ,  \"τ1\" -> 0.181870145043   ,  \"τS\" -> 0.168113301561   ,  \"τN\" -> 0.186965229666   ,  \"τC\" -> 0.001543998203   ,  \"κ0\" -> 0.000000000530   ,  \"mm1\" -> 0.000318362571   ,  \"mm2\" -> 0.069029342513   ,  \"mm3\" -> 0.562051433928   ,  \"T\" -> 0.122000000000   ,  \"B\" -> 8.000000000000   ,  \"θ\" -> 0.000000000000   ,  \"Reoff\" -> -63674698.795180723100   ,  \"Imoff\" -> 0.000000000000    |>   , \r\"IDS0379_210909_RAW_cal__ref_\" ->   <|    \"ζ\" -> 0.361462767147   ,  \"τ1\" -> 0.107500538930   ,  \"τS\" -> 0.062213194344   ,  \"τN\" -> 0.084141320306   ,  \"τC\" -> 0.001080078747   ,  \"κ0\" -> 0.000000000626   ,  \"mm1\" -> 0.000284077168   ,  \"mm2\" -> 0.033543691937   ,  \"mm3\" -> 0.274009071072   ,  \"T\" -> 0.148000000000   ,  \"B\" -> 8.000000000000   ,  \"θ\" -> 0.000000000000   ,  \"Reoff\" -> -69828313.253012046200   ,  \"Imoff\" -> 0.000000000000    |>   , \r\"IDS0379_210909_RAW_cal__sam_\" ->   <|    \"ζ\" -> 0.225699737863   ,  \"τ1\" -> 0.105340283181   ,  \"τS\" -> 0.080581728797   ,  \"τN\" -> 0.103261234048   ,  \"τC\" -> 0.001367459466   ,  \"κ0\" -> 0.000000000745   ,  \"mm1\" -> 0.000248975261   ,  \"mm2\" -> 0.035515573270   ,  \"mm3\" -> 0.296279465482   ,  \"T\" -> 0.148000000000   ,  \"B\" -> 8.000000000000   ,  \"θ\" -> 0.000000000000   ,  \"Reoff\" -> -47870481.927710846100   ,  \"Imoff\" -> 0.000000000000    |>   , \r\"IDS0380_210909_RAW_cal__ref_\" ->   <|    \"ζ\" -> 0.284519772107   ,  \"τ1\" -> 0.082886192682   ,  \"τS\" -> 0.042651392468   ,  \"τN\" -> 0.053095048754   ,  \"τC\" -> 0.001034420795   ,  \"κ0\" -> 0.000000000747   ,  \"mm1\" -> 0.000225779274   ,  \"mm2\" -> 0.025423829331   ,  \"mm3\" -> 0.181259201730   ,  \"T\" -> 0.168000000000   ,  \"B\" -> 8.000000000000   ,  \"θ\" -> 0.000000000000   ,  \"Reoff\" -> -49656626.506024099900   ,  \"Imoff\" -> 0.000000000000    |>   , \r\"IDS0380_210909_RAW_cal__sam_\" ->   <|    \"ζ\" -> 0.175751625392   ,  \"τ1\" -> 0.093635045165   ,  \"τS\" -> 0.061160146348   ,  \"τN\" -> 0.068664853746   ,  \"τC\" -> 0.001317909381   ,  \"κ0\" -> 0.000000000855   ,  \"mm1\" -> 0.000193962663   ,  \"mm2\" -> 0.031705338902   ,  \"mm3\" -> 0.215695607858   ,  \"T\" -> 0.168000000000   ,  \"B\" -> 8.000000000000   ,  \"θ\" -> 0.000000000000   ,  \"Reoff\" -> -37527108.433734938500   ,  \"Imoff\" -> 0.000000000000    |>   , \r\"IDS0381_210909_RAW_cal__ref_\" ->   <|    \"ζ\" -> 0.127050352056   ,  \"τ1\" -> 0.057128460751   ,  \"τS\" -> 0.026895519029   ,  \"τN\" -> 0.010742183960   ,  \"τC\" -> 0.001220655243   ,  \"κ0\" -> 0.000000001351   ,  \"mm1\" -> 0.000132830935   ,  \"mm2\" -> 0.023152174040   ,  \"mm3\" -> 0.077483697423   ,  \"T\" -> 0.250000000000   ,  \"B\" -> 8.000000000000   ,  \"θ\" -> 0.000000000000   ,  \"Reoff\" -> -15819277.108433738400   ,  \"Imoff\" -> 0.000000000000    |>   , \r\"IDS0381_210909_RAW_cal__sam_\" ->   <|    \"ζ\" -> 0.077362618852   ,  \"τ1\" -> 0.058638638627   ,  \"τS\" -> 0.035602410157   ,  \"τN\" -> 0.012932252536   ,  \"τC\" -> 0.001722606032   ,  \"κ0\" -> 0.000000001497   ,  \"mm1\" -> 0.000118727642   ,  \"mm2\" -> 0.027585733079   ,  \"mm3\" -> 0.084946215242   ,  \"T\" -> 0.250000000000   ,  \"B\" -> 8.000000000000   ,  \"θ\" -> 0.000000000000   ,  \"Reoff\" -> -9843373.493975907570   ,  \"Imoff\" -> 0.000000000000    |>   , \r\"IDS0382_210909_RAW_cal__ref_\" ->   <|    \"ζ\" -> 0.087791328975   ,  \"τ1\" -> 0.049440394886   ,  \"τS\" -> 0.024402785598   ,  \"τN\" -> 0.005535568337   ,  \"τC\" -> 0.001508144089   ,  \"κ0\" -> 0.000000001731   ,  \"mm1\" -> 0.000115646552   ,  \"mm2\" -> 0.022789793756   ,  \"mm3\" -> 0.060609780481   ,  \"T\" -> 0.300000000000   ,  \"B\" -> 8.000000000000   ,  \"θ\" -> 0.000000000000   ,  \"Reoff\" -> -8144578.313253011560   ,  \"Imoff\" -> 0.000000000000    |>   , \r\"IDS0382_210909_RAW_cal__sam_\" ->   <|    \"ζ\" -> 0.054029770351   ,  \"τ1\" -> 0.051440847518   ,  \"τS\" -> 0.032079834642   ,  \"τN\" -> 0.007150632998   ,  \"τC\" -> 0.002202148776   ,  \"κ0\" -> 0.000000001884   ,  \"mm1\" -> 0.000106291219   ,  \"mm2\" -> 0.027352636275   ,  \"mm3\" -> 0.067534149597   ,  \"T\" -> 0.300000000000   ,  \"B\" -> 8.000000000000   ,  \"θ\" -> 0.000000000000   ,  \"Reoff\" -> 0.000000000000   ,  \"Imoff\" -> 0.000000000000    |>   , \r\"IDS0383_210910_RAW_cal__ref_\" ->   <|    \"ζ\" -> 0.062586766538   ,  \"τ1\" -> 0.048322657274   ,  \"τS\" -> 0.023582446152   ,  \"τN\" -> 0.003596780616   ,  \"τC\" -> 0.001965770478   ,  \"κ0\" -> 0.000000002106   ,  \"mm1\" -> 0.000107789725   ,  \"mm2\" -> 0.023345406911   ,  \"mm3\" -> 0.055715517805   ,  \"T\" -> 0.360000000000   ,  \"B\" -> 8.000000000000   ,  \"θ\" -> 0.000000000000   ,  \"Reoff\" -> 0.000000000000   ,  \"Imoff\" -> 0.000000000000    |>   , \r\"IDS0383_210910_RAW_cal__sam_\" ->   <|    \"ζ\" -> 0.038341835326   ,  \"τ1\" -> 0.050866858713   ,  \"τS\" -> 0.030652081909   ,  \"τN\" -> 0.004623805952   ,  \"τC\" -> 0.002823684758   ,  \"κ0\" -> 0.000000002289   ,  \"mm1\" -> 0.000096034779   ,  \"mm2\" -> 0.028459102290   ,  \"mm3\" -> 0.061763836547   ,  \"T\" -> 0.360000000000   ,  \"B\" -> 8.000000000000   ,  \"θ\" -> 0.000000000000   ,  \"Reoff\" -> 0.000000000000   ,  \"Imoff\" -> 0.000000000000    |>   , \r\"IDS0384_210910_RAW_cal__ref_\" ->   <|    \"ζ\" -> 0.047320664202   ,  \"τ1\" -> 0.050730770684   ,  \"τS\" -> 0.023716512211   ,  \"τN\" -> 0.002200072160   ,  \"τC\" -> 0.002249629457   ,  \"κ0\" -> 0.000000002636   ,  \"mm1\" -> 0.000093524415   ,  \"mm2\" -> 0.024793115562   ,  \"mm3\" -> 0.055236734521   ,  \"T\" -> 0.430000000000   ,  \"B\" -> 8.000000000000   ,  \"θ\" -> 0.000000000000   ,  \"Reoff\" -> 0.000000000000   ,  \"Imoff\" -> 0.000000000000    |>   , \r\"IDS0384_210910_RAW_cal__sam_\" ->   <|    \"ζ\" -> 0.029950572027   ,  \"τ1\" -> 0.044923259835   ,  \"τS\" -> 0.030416367718   ,  \"τN\" -> 0.002541256331   ,  \"τC\" -> 0.003331031560   ,  \"κ0\" -> 0.000000002858   ,  \"mm1\" -> 0.000087776347   ,  \"mm2\" -> 0.029544080465   ,  \"mm3\" -> 0.052567158325   ,  \"T\" -> 0.430000000000   ,  \"B\" -> 8.000000000000   ,  \"θ\" -> 0.000000000000   ,  \"Reoff\" -> 0.000000000000   ,  \"Imoff\" -> 0.000000000000    |>   , \r\"IDS0385_210910_RAW_cal__ref_\" ->   <|    \"ζ\" -> 0.037147896010   ,  \"τ1\" -> 0.047226564206   ,  \"τS\" -> 0.024619467421   ,  \"τN\" -> 0.001310789285   ,  \"τC\" -> 0.002565709752   ,  \"κ0\" -> 0.000000003275   ,  \"mm1\" -> 0.000083755028   ,  \"mm2\" -> 0.026306932368   ,  \"mm3\" -> 0.050295097748   ,  \"T\" -> 0.530000000000   ,  \"B\" -> 8.000000000000   ,  \"θ\" -> 0.000000000000   ,  \"Reoff\" -> 0.000000000000   ,  \"Imoff\" -> 0.000000000000    |>   , \r\"IDS0385_210910_RAW_cal__sam_\" ->   <|    \"ζ\" -> 0.024600756648   ,  \"τ1\" -> 0.043958236582   ,  \"τS\" -> 0.031312750224   ,  \"τN\" -> 0.001348105931   ,  \"τC\" -> 0.003635120795   ,  \"κ0\" -> 0.000000003548   ,  \"mm1\" -> 0.000078569164   ,  \"mm2\" -> 0.031960914170   ,  \"mm3\" -> 0.049018211972   ,  \"T\" -> 0.530000000000   ,  \"B\" -> 8.000000000000   ,  \"θ\" -> 0.000000000000   ,  \"Reoff\" -> 0.000000000000   ,  \"Imoff\" -> 0.000000000000    |>   , \r\"IDS0386_210910_RAW_cal__ref_\" ->   <|    \"ζ\" -> 0.028995432115   ,  \"τ1\" -> 0.046559455187   ,  \"τS\" -> 0.026126949833   ,  \"τN\" -> 0.000676599034   ,  \"τC\" -> 0.003300199116   ,  \"κ0\" -> 0.000000003897   ,  \"mm1\" -> 0.000083055023   ,  \"mm2\" -> 0.028956759593   ,  \"mm3\" -> 0.048400569036   ,  \"T\" -> 0.630000000000   ,  \"B\" -> 8.000000000000   ,  \"θ\" -> 0.000000000000   ,  \"Reoff\" -> 0.000000000000   ,  \"Imoff\" -> 0.000000000000    |>   , \r\"IDS0386_210910_RAW_cal__sam_\" ->   <|    \"ζ\" -> 0.019494767421   ,  \"τ1\" -> 0.040349410363   ,  \"τS\" -> 0.033202805363   ,  \"τN\" -> 0.000770756985   ,  \"τC\" -> 0.004303152006   ,  \"κ0\" -> 0.000000004241   ,  \"mm1\" -> 0.000073144130   ,  \"mm2\" -> 0.033928832906   ,  \"mm3\" -> 0.045286454378   ,  \"T\" -> 0.630000000000   ,  \"B\" -> 8.000000000000   ,  \"θ\" -> 0.000000000000   ,  \"Reoff\" -> 0.000000000000   ,  \"Imoff\" -> 0.000000000000    |>   , \r\"IDS0387_210910_RAW_cal__ref_\" ->   <|    \"ζ\" -> 0.021158107821   ,  \"τ1\" -> 0.047181877660   ,  \"τS\" -> 0.030519366684   ,  \"τN\" -> 0.000257878410   ,  \"τC\" -> 0.004211881541   ,  \"κ0\" -> 0.000000005418   ,  \"mm1\" -> 0.000077046675   ,  \"mm2\" -> 0.034577725836   ,  \"mm3\" -> 0.048167420054   ,  \"T\" -> 0.830000000000   ,  \"B\" -> 8.000000000000   ,  \"θ\" -> 0.000000000000   ,  \"Reoff\" -> 0.000000000000   ,  \"Imoff\" -> 0.000000000000    |>   , \r\"IDS0387_210910_RAW_cal__sam_\" ->   <|    \"ζ\" -> 0.013958531253   ,  \"τ1\" -> 0.040449551738   ,  \"τS\" -> 0.038075316972   ,  \"τN\" -> 0.000218997482   ,  \"τC\" -> 0.005348147372   ,  \"κ0\" -> 0.000000005866   ,  \"mm1\" -> 0.000064761782   ,  \"mm2\" -> 0.038768935960   ,  \"mm3\" -> 0.045792848207   ,  \"T\" -> 0.830000000000   ,  \"B\" -> 8.000000000000   ,  \"θ\" -> 0.000000000000   ,  \"Reoff\" -> 0.000000000000   ,  \"Imoff\" -> 0.000000000000    |>   , \r\"IDS0388_210910_RAW_cal__ref_\" ->   <|    \"ζ\" -> 0.017074092265   ,  \"τ1\" -> 0.047215899415   ,  \"τS\" -> 0.039490388664   ,  \"τN\" -> 0.000122819272   ,  \"τC\" -> 0.004722965607   ,  \"κ0\" -> 0.000000007547   ,  \"mm1\" -> 0.000071056708   ,  \"mm2\" -> 0.043397222666   ,  \"mm3\" -> 0.048760153151   ,  \"T\" -> 1.130000000000   ,  \"B\" -> 8.000000000000   ,  \"θ\" -> 0.000000000000   ,  \"Reoff\" -> 0.000000000000   ,  \"Imoff\" -> 0.000000000000    |>   , \r\"IDS0388_210910_RAW_cal__sam_\" ->   <|    \"ζ\" -> 0.011551866824   ,  \"τ1\" -> 0.040411227639   ,  \"τS\" -> 0.048181354691   ,  \"τN\" -> 0.000103559724   ,  \"τC\" -> 0.006232382617   ,  \"κ0\" -> 0.000000008161   ,  \"mm1\" -> 0.000063176601   ,  \"mm2\" -> 0.040126882627   ,  \"mm3\" -> 0.055296246344   ,  \"T\" -> 1.130000000000   ,  \"B\" -> 8.000000000000   ,  \"θ\" -> 0.000000000000   ,  \"Reoff\" -> 0.000000000000   ,  \"Imoff\" -> 0.000000000000    |>   , \r\"IDS0389_210910_RAW_cal__ref_\" ->   <|    \"ζ\" -> 0.017157539727   ,  \"τ1\" -> 0.046379456311   ,  \"τS\" -> 0.015264158508   ,  \"τN\" -> 0.000057006071   ,  \"τC\" -> 0.004702188691   ,  \"κ0\" -> 0.000000010470   ,  \"mm1\" -> 0.000061063584   ,  \"mm2\" -> 0.020122781068   ,  \"mm3\" -> 0.046481838419   ,  \"T\" -> 1.520000000000   ,  \"B\" -> 8.000000000000   ,  \"θ\" -> 0.000000000000   ,  \"Reoff\" -> 0.000000000000   ,  \"Imoff\" -> 0.000000000000    |>   , \r\"IDS0389_210910_RAW_cal__sam_\" ->   <|    \"ζ\" -> 0.011148198813   ,  \"τ1\" -> 0.038849151842   ,  \"τS\" -> 0.019213865355   ,  \"τN\" -> 0.000045035153   ,  \"τC\" -> 0.005536708133   ,  \"κ0\" -> 0.000000011229   ,  \"mm1\" -> 0.000047596165   ,  \"mm2\" -> 0.024836509281   ,  \"mm3\" -> 0.038975357089   ,  \"T\" -> 1.520000000000   ,  \"B\" -> 8.000000000000   ,  \"θ\" -> 0.000000000000   ,  \"Reoff\" -> 0.000000000000   ,  \"Imoff\" -> 0.000000000000    |>   , \r\"IDS0390_210910_RAW_cal__ref_\" ->   <|    \"ζ\" -> 0.016425367394   ,  \"τ1\" -> 0.039829137916   ,  \"τS\" -> 0.010121167967   ,  \"τN\" -> 0.000033814494   ,  \"τC\" -> 0.004533563026   ,  \"κ0\" -> 0.000000013089   ,  \"mm1\" -> 0.000051027686   ,  \"mm2\" -> 0.014749763975   ,  \"mm3\" -> 0.039883691060   ,  \"T\" -> 1.900000000000   ,  \"B\" -> 8.000000000000   ,  \"θ\" -> 0.000000000000   ,  \"Reoff\" -> 0.000000000000   ,  \"Imoff\" -> 0.000000000000    |>   , \r\"IDS0390_210910_RAW_cal__sam_\" ->   <|    \"ζ\" -> 0.010826949430   ,  \"τ1\" -> 0.038768037521   ,  \"τS\" -> 0.012925317198   ,  \"τN\" -> 0.000029157336   ,  \"τC\" -> 0.005196063884   ,  \"κ0\" -> 0.000000013864   ,  \"mm1\" -> 0.000039906108   ,  \"mm2\" -> 0.018195372076   ,  \"mm3\" -> 0.038823555195   ,  \"T\" -> 1.900000000000   ,  \"B\" -> 8.000000000000   ,  \"θ\" -> 0.000000000000   ,  \"Reoff\" -> 0.000000000000   ,  \"Imoff\" -> 0.000000000000    |>   , \r\"IDS0391_210910_RAW_cal__ref_\" ->   <|    \"ζ\" -> 0.016160769926   ,  \"τ1\" -> 0.047360928893   ,  \"τS\" -> 0.041725389227   ,  \"τN\" -> 0.000076715950   ,  \"τC\" -> 0.004871049589   ,  \"κ0\" -> 0.000000008346   ,  \"mm1\" -> 0.000069587647   ,  \"mm2\" -> 0.045398277439   ,  \"mm3\" -> 0.049241772777   ,  \"T\" -> 1.250000000000   ,  \"B\" -> 8.000000000000   ,  \"θ\" -> 0.000000000000   ,  \"Reoff\" -> 0.000000000000   ,  \"Imoff\" -> 0.000000000000    |>   , \r\"IDS0391_210910_RAW_cal__sam_\" ->   <|    \"ζ\" -> 0.010962610928   ,  \"τ1\" -> 0.040398807374   ,  \"τS\" -> 0.051328988590   ,  \"τN\" -> 0.000070281011   ,  \"τC\" -> 0.006422533164   ,  \"κ0\" -> 0.000000008958   ,  \"mm1\" -> 0.000062039854   ,  \"mm2\" -> 0.040240103995   ,  \"mm3\" -> 0.058481936484   ,  \"T\" -> 1.250000000000   ,  \"B\" -> 8.000000000000   ,  \"θ\" -> 0.000000000000   ,  \"Reoff\" -> 0.000000000000   ,  \"Imoff\" -> 0.000000000000    |>   , \r\"IDS0392_210910_RAW_cal__ref_\" ->   <|    \"ζ\" -> 0.016250541117   ,  \"τ1\" -> 0.047393343666   ,  \"τS\" -> 0.029998719281   ,  \"τN\" -> 0.000076850447   ,  \"τC\" -> 0.004810494325   ,  \"κ0\" -> 0.000000009475   ,  \"mm1\" -> 0.000066564951   ,  \"mm2\" -> 0.035009422265   ,  \"mm3\" -> 0.047692164786   ,  \"T\" -> 1.390000000000   ,  \"B\" -> 8.000000000000   ,  \"θ\" -> 0.000000000000   ,  \"Reoff\" -> 0.000000000000   ,  \"Imoff\" -> 0.000000000000    |>   , \r\"IDS0392_210910_RAW_cal__sam_\" ->   <|    \"ζ\" -> 0.010962610928   ,  \"τ1\" -> 0.040398807374   ,  \"τS\" -> 0.051328988590   ,  \"τN\" -> 0.000070281011   ,  \"τC\" -> 0.006422533164   ,  \"κ0\" -> 0.000000008958   ,  \"mm1\" -> 0.000062039854   ,  \"mm2\" -> 0.040240103995   ,  \"mm3\" -> 0.058481936484   ,  \"T\" -> 1.390000000000   ,  \"B\" -> 8.000000000000   ,  \"θ\" -> 0.000000000000   ,  \"Reoff\" -> 0.000000000000   ,  \"Imoff\" -> 0.000000000000    |>   , \r\"IDS0393_210910_RAW_cal__ref_\" ->   <|    \"ζ\" -> 0.015227705493   ,  \"τ1\" -> 0.038797003927   ,  \"τS\" -> 0.007286355621   ,  \"τN\" -> 0.000013994204   ,  \"τC\" -> 0.003959851165   ,  \"κ0\" -> 0.000000023455   ,  \"mm1\" -> 0.000038818663   ,  \"mm2\" -> 0.011312505580   ,  \"mm3\" -> 0.038817048251   ,  \"T\" -> 3.110000000000   ,  \"B\" -> 8.000000000000   ,  \"θ\" -> 0.000000000000   ,  \"Reoff\" -> 0.000000000000   ,  \"Imoff\" -> 0.000000000000    |>   , \r\"IDS0393_210910_RAW_cal__sam_\" ->   <|    \"ζ\" -> 0.010962610928   ,  \"τ1\" -> 0.040398807374   ,  \"τS\" -> 0.051328988590   ,  \"τN\" -> 0.000070281011   ,  \"τC\" -> 0.006422533164   ,  \"κ0\" -> 0.000000008958   ,  \"mm1\" -> 0.000062039854   ,  \"mm2\" -> 0.040240103995   ,  \"mm3\" -> 0.058481936484   ,  \"T\" -> 3.110000000000   ,  \"B\" -> 8.000000000000   ,  \"θ\" -> 0.000000000000   ,  \"Reoff\" -> 0.000000000000   ,  \"Imoff\" -> 0.000000000000    |>   , \r\"IDS0394_210910_RAW_cal__ref_\" ->   <|    \"ζ\" -> 0.018884017265   ,  \"τ1\" -> 0.038756536887   ,  \"τS\" -> 0.005123025136   ,  \"τN\" -> 0.000004793994   ,  \"τC\" -> 0.002621800478   ,  \"κ0\" -> 0.000000058143   ,  \"mm1\" -> 0.000032480301   ,  \"mm2\" -> 0.007807858865   ,  \"mm3\" -> 0.038762651153   ,  \"T\" -> 5.750000000000   ,  \"B\" -> 8.000000000000   ,  \"θ\" -> 0.000000000000   ,  \"Reoff\" -> 0.000000000000   ,  \"Imoff\" -> 0.000000000000    |>   , \r\"IDS0394_210910_RAW_cal__sam_\" ->   <|    \"ζ\" -> 0.010962610928   ,  \"τ1\" -> 0.040398807374   ,  \"τS\" -> 0.051328988590   ,  \"τN\" -> 0.000070281011   ,  \"τC\" -> 0.006422533164   ,  \"κ0\" -> 0.000000008958   ,  \"mm1\" -> 0.000062039854   ,  \"mm2\" -> 0.040240103995   ,  \"mm3\" -> 0.058481936484   ,  \"T\" -> 5.750000000000   ,  \"B\" -> 8.000000000000   ,  \"θ\" -> 0.000000000000   ,  \"Reoff\" -> 0.000000000000   ,  \"Imoff\" -> 0.000000000000    |>   , \r\"IDS0395_210910_RAW_cal__ref_\" ->   <|    \"ζ\" -> 0.016101273075   ,  \"τ1\" -> 0.047373144247   ,  \"τS\" -> 0.040453117489   ,  \"τN\" -> 0.000076678480   ,  \"τC\" -> 0.005036745304   ,  \"κ0\" -> 0.000000008627   ,  \"mm1\" -> 0.000071210472   ,  \"mm2\" -> 0.044744190963   ,  \"mm3\" -> 0.048776865397   ,  \"T\" -> 1.310000000000   ,  \"B\" -> 8.000000000000   ,  \"θ\" -> 0.000000000000   ,  \"Reoff\" -> 0.000000000000   ,  \"Imoff\" -> 0.000000000000    |>   , \r\"IDS0395_210910_RAW_cal__sam_\" ->   <|    \"ζ\" -> 0.010962610928   ,  \"τ1\" -> 0.040398807374   ,  \"τS\" -> 0.051328988590   ,  \"τN\" -> 0.000070281011   ,  \"τC\" -> 0.006422533164   ,  \"κ0\" -> 0.000000008958   ,  \"mm1\" -> 0.000062039854   ,  \"mm2\" -> 0.040240103995   ,  \"mm3\" -> 0.058481936484   ,  \"T\" -> 1.310000000000   ,  \"B\" -> 8.000000000000   ,  \"θ\" -> 0.000000000000   ,  \"Reoff\" -> 0.000000000000   ,  \"Imoff\" -> 0.000000000000    |>   , \r"
  in  "Math→ string OUT! :s":bool
  in  "string IN → Math!":bool
  in  "file pattern":string="IDS*RAW*_raw_.dat"
  in  "folder":path=path "/opt/new/Dropbox/shared_AkashAndreas/paper-CeCoIn5/Original RAW data"
